vi "Main.vi"() -> ()   [LabVIEW 2013]
uses:
  <vilib>/vision/Image Controls.llb/IMAQ Image.ctl
  <vilib>/Instr/_visa.llb/VISA Flush IO Buffer Mask.ctl
  <vilib>/Instr/_visa.llb/VISA Configure Serial Port (Instr).vi
  <vilib>/vision/NI_Vision_Development_Module.lvlib
panel:
  out "Original Heading Image":T1
  out "Roll Array":dbl[](array[numeric])
  out "Pitch Array":dbl[](array[numeric])
  out "Time for Orientation":dbl[](array[numeric])
  out "Time for Temp":dbl[](array[numeric])
  out "Heater Temp":dbl[](array[numeric])
  out "Temp 2":dbl[](array[numeric])
  out "Temp 1":dbl[](array[numeric])
  out "Start time (minutes)":dbl
  out "error out":errorcluster
  in  "error in (no error)":errorcluster
  in  "Tab Control":T2(tab)
  in  "Yaw":dbl(slide) scale=-180.0..180.0
  in  "Roll":dbl(slide) scale=-10.0..10.0
  in  "Pitch":dbl(slide) scale=-10.0..10.0
  out "Manual Heat Control?":bool
  out "Current Time":timestamp format="%<%I:%M:%S %p>T"
  in  "Command":u16(ring) items=["CUTDOWN"=0, "CHANGE_TRANSMIT_RATE"=1, "TURN_HEATER_ON"=2, "TURN_HEATER_OFF"=3, "MANUAL_HEATER_CONTROL"=4, "GET_INTERIOR_TEMP"=16534, "GET_EXTERIOR_TEMP"=16535, "GET_PRESSURE"=16536, "GET_HUMIDITY"=16537, "GET_PITCH"=16640, "GET_ROLL"=16641, "GET_YAW"=16642, "GET_HEATER_STATUS"=16643]
  in  "Value":u16
  out "Sensor Specifications Exceeded":bool caption="Warning"
  in  "Stop":bool
  in  "Last Recieved Packet":string
  out "Radio Connection Lost":bool caption="Alarm"
  out "Turbulence":bool caption="Warning"
  out "Success?":bool
  in  "Baud Rate":i32=115200
  out "Data Logging OFF":bool caption="Warning"
  in  "Packet Logging File":path
  in  "Log Recieved Packets?":bool=TRUE
  out "Time of Last Recieved Packet":timestamp format="%<%I:%M:%S %p>T"
  out "Heater On?":bool
  out "Yaw":dbl
  out "Roll":dbl
  out "Pitch":dbl
  in  "COM Port":refnum<visa-resource-name>
  in  "Send Command":bool
  out "Response":string
  in  "Interior Temperature 2":dbl(knob) scale=-60.0..40.0
  out "Yaw":T1(plugin-control)
  out "Pitch":dbl(slide) scale=-25.0..25.0
  out "Roll":dbl(slide) scale=-25.0..25.0
  out "Relative Humidity":dbl(knob) scale=0.0..100.0
  out "Atmospheric Pressure":dbl(knob) scale=0.0..15.0
  out "Flight Duration":timestamp format="%<%H:%M:%S>T"
  out "Low Interior Temperature":bool caption="Warning"
  out "Critically Low Interior Temperature":bool caption="Alarm"
  in  "Interior Temperature 1":dbl(knob) scale=-60.0..40.0
  in  "Exterior Temperature":dbl(knob) scale=-60.0..40.0
  in  "Heater Temperature":dbl(knob) scale=-60.0..40.0
  out "Yaw":cluster{"X":dbl, "Y":dbl}[](graph)
  out "Atmospheric Pressure":cluster{"X":dbl, "Y":dbl}[](graph)
  out "Exterior Temperature":cluster{"X":dbl, "Y":dbl}[](graph)
  out "Relative Humidity":cluster{"X":dbl, "Y":dbl}[](graph)
  out "Interior Temperature":cluster{dbl[], dbl[]}[](graph)
  out "Pitch/Roll":cluster{dbl[], dbl[]}[](graph)
  in  "Save Packets":bool
  in  "Packet File":path
  out "Packets Recieved":string
  # "Current Instrument Readings"
  # "Orientation"
  # "Control"
  # "Warnings and Alarms"
  # "Communication"
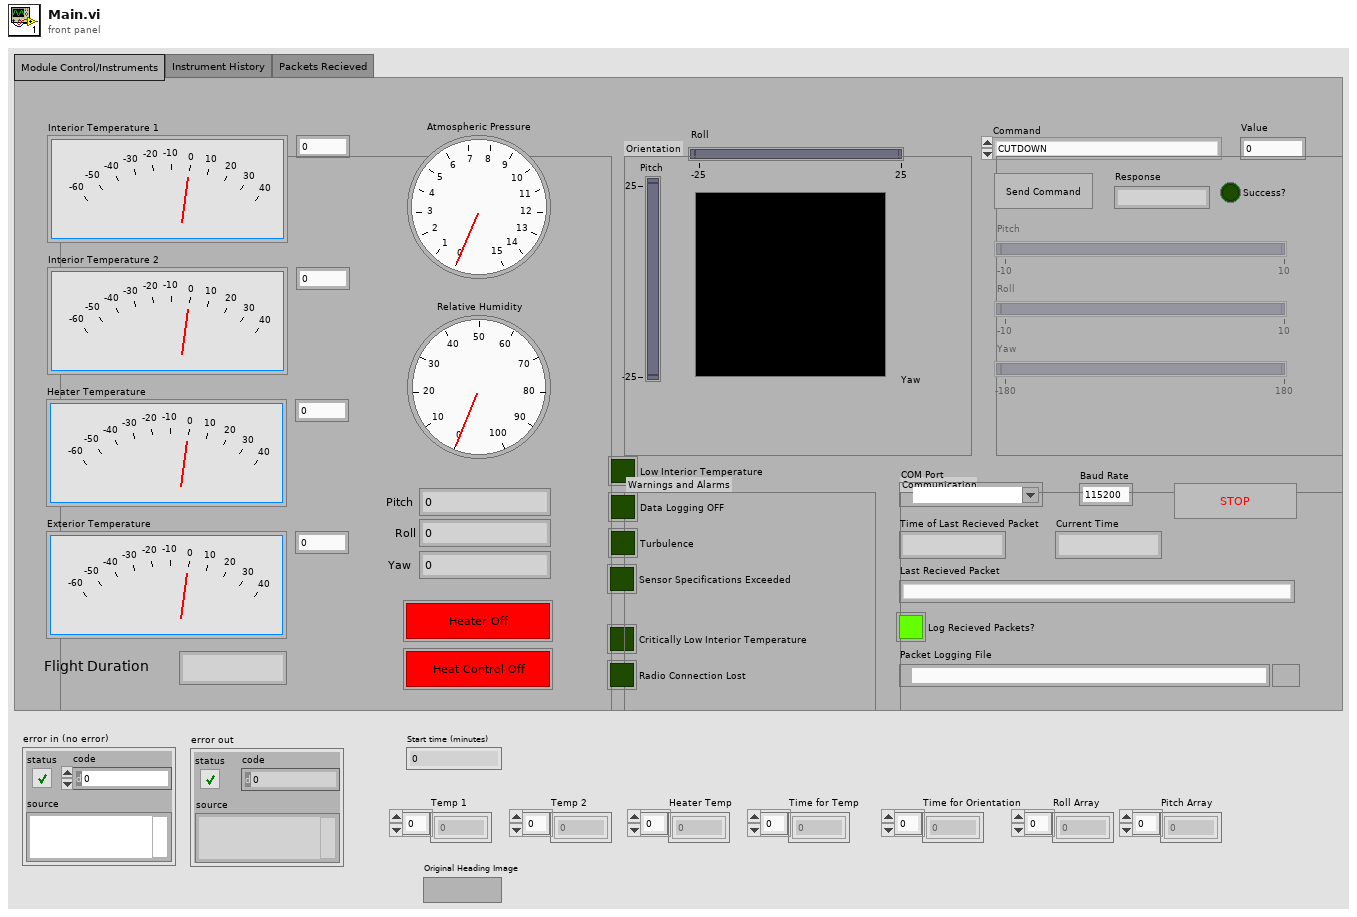
[diagram p1: front panel]
types:
  T1 = typedef "IMAQ Image.ctl" = refnum<image>
  T2 = enum32{"Module Control/Instruments", "Instrument History", "Packets Recieved"}
  T3 = typedef "VISA Flush IO Buffer Mask.ctl" = u16
  T4 = enum16{"open", "replace", "create", "open or create", "replace or create", "replace or create with confirmation"}
  T5 = cluster{"Blue or Luma":u8, "Green or Sat Plane":u8, "Red or Hue Plane":u8, "Alpha":u8}
  T6 = cluster{"Digital Interior Temperature":dbl, "Analog Interior Temperature":dbl, "Heater Temperature":dbl, "Exterior Temperature":dbl, "Humidity":dbl, "Pressure":dbl, "Pitch":dbl, "Roll":dbl, "Yaw":dbl, "Heater On?":bool, "Data Logging?":bool, "Manual Heat Control?":bool, "Turbulence":bool}
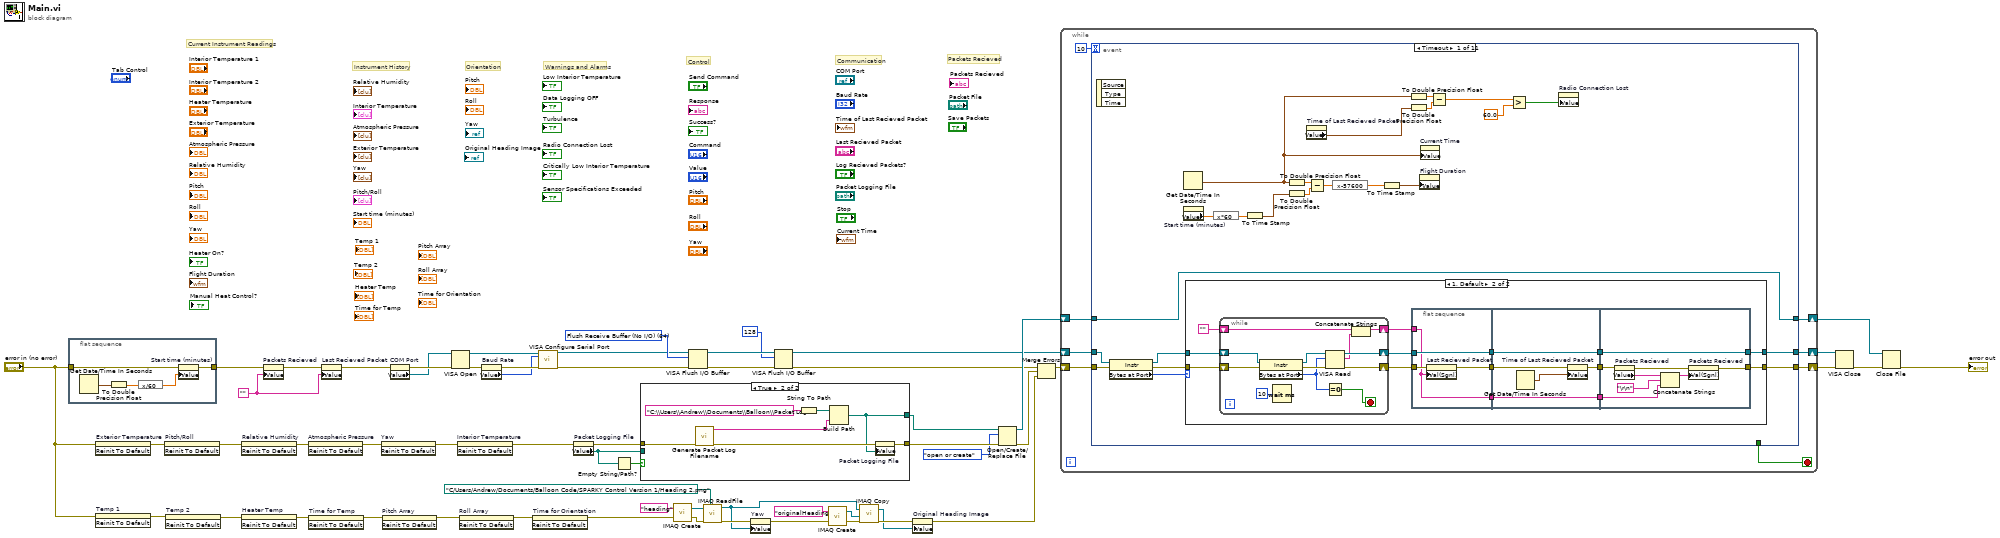
[diagram p0: block diagram]
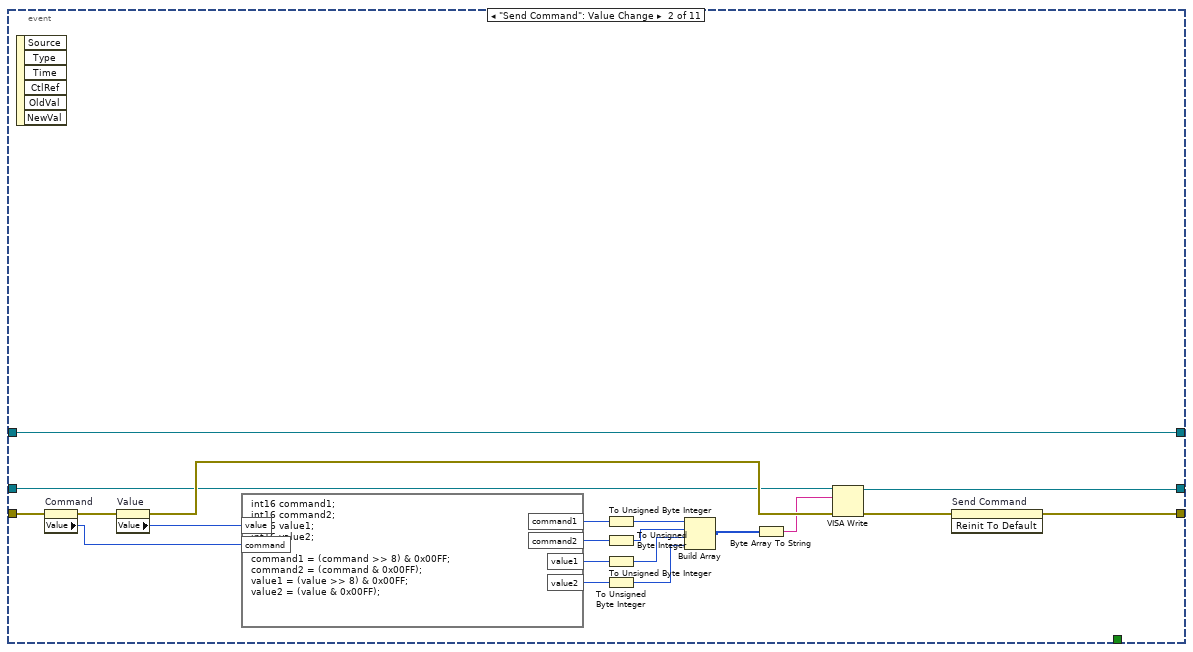
[diagram p4: hidden frame]
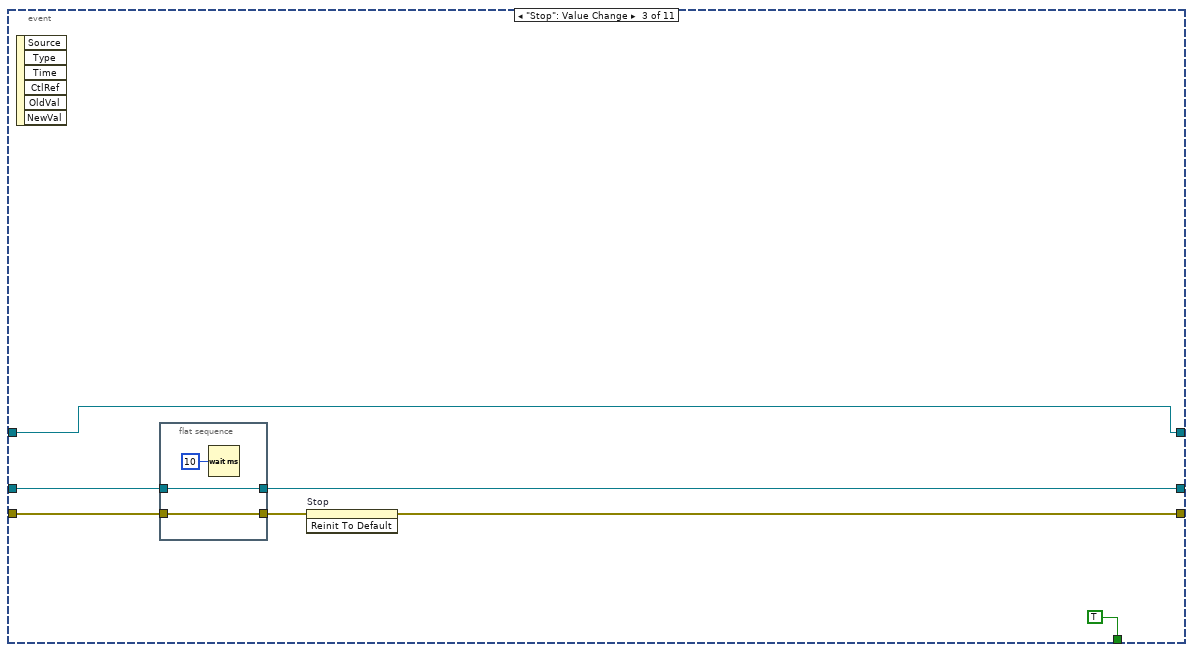
[diagram p5: hidden frame]
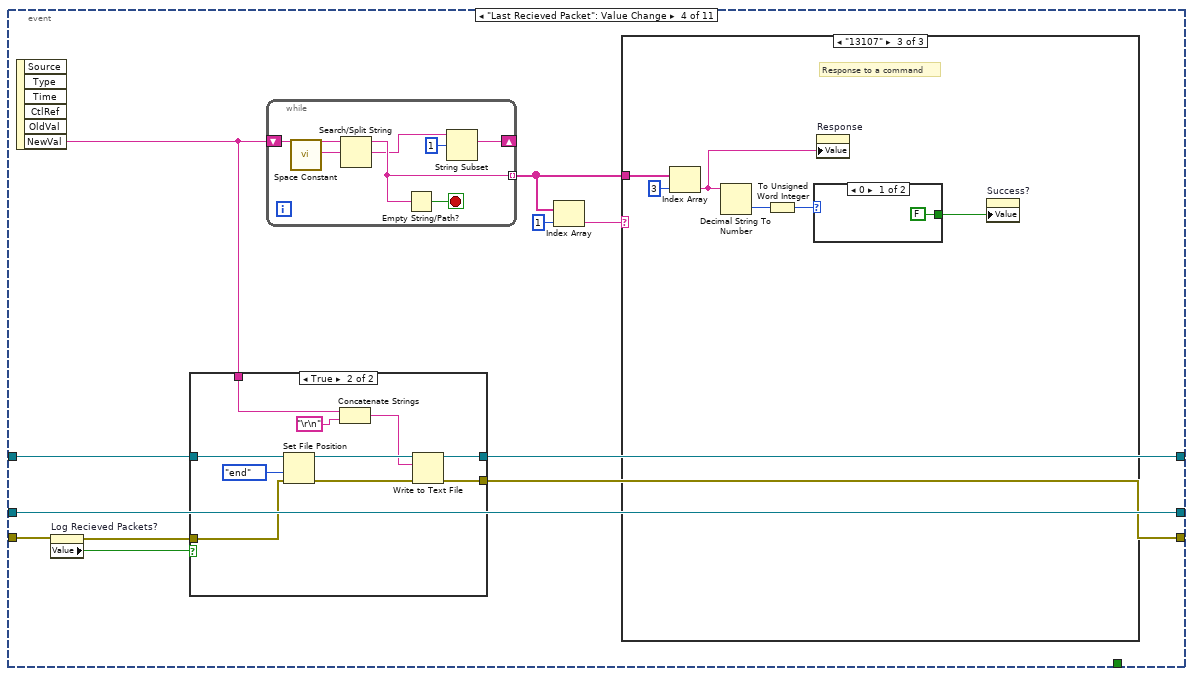
[diagram p6: hidden frame]
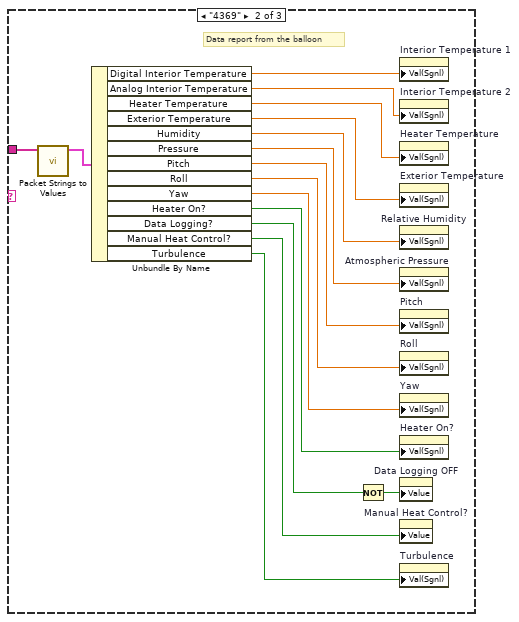
[diagram p8: hidden frame]
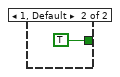
[diagram p9: hidden frame]
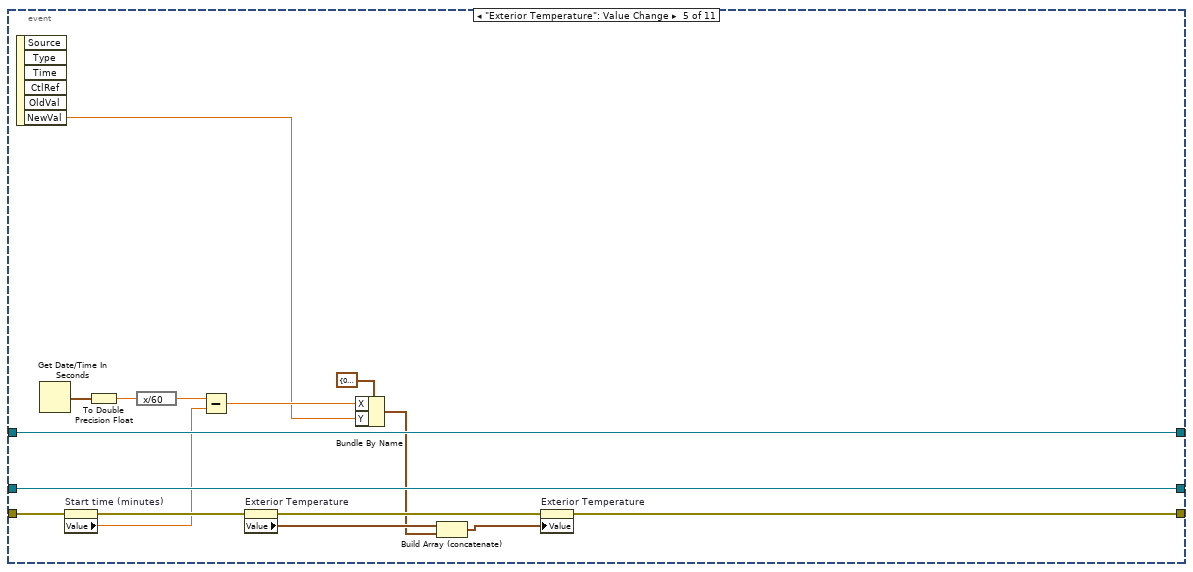
[diagram p11: hidden frame]
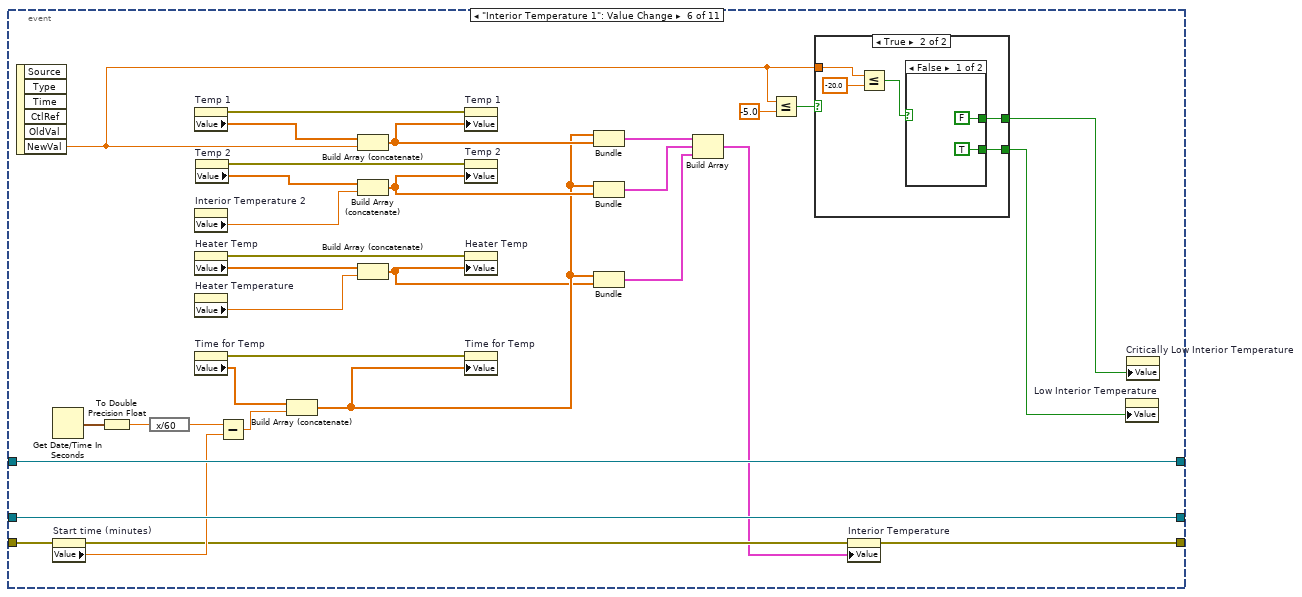
[diagram p12: hidden frame]
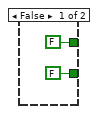
[diagram p13: hidden frame]
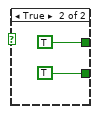
[diagram p14: hidden frame]
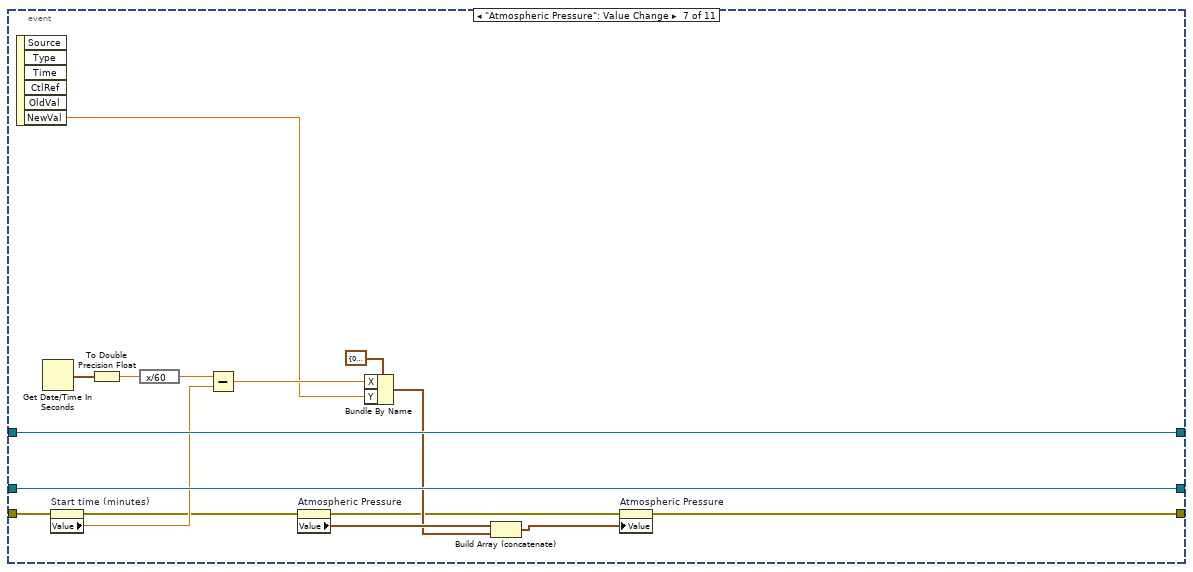
[diagram p15: hidden frame]
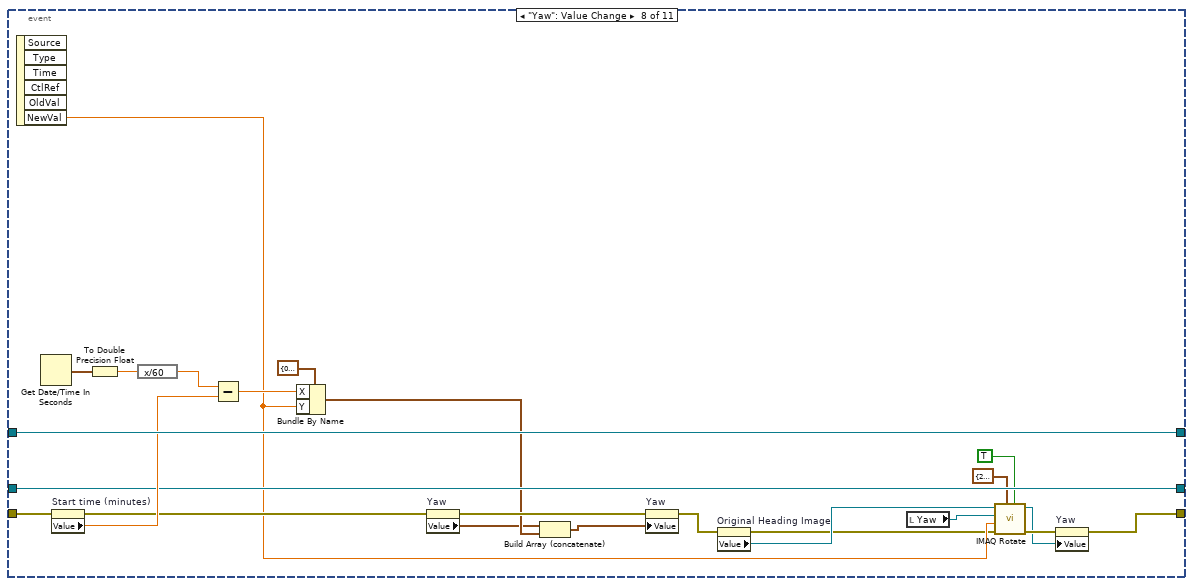
[diagram p16: hidden frame]
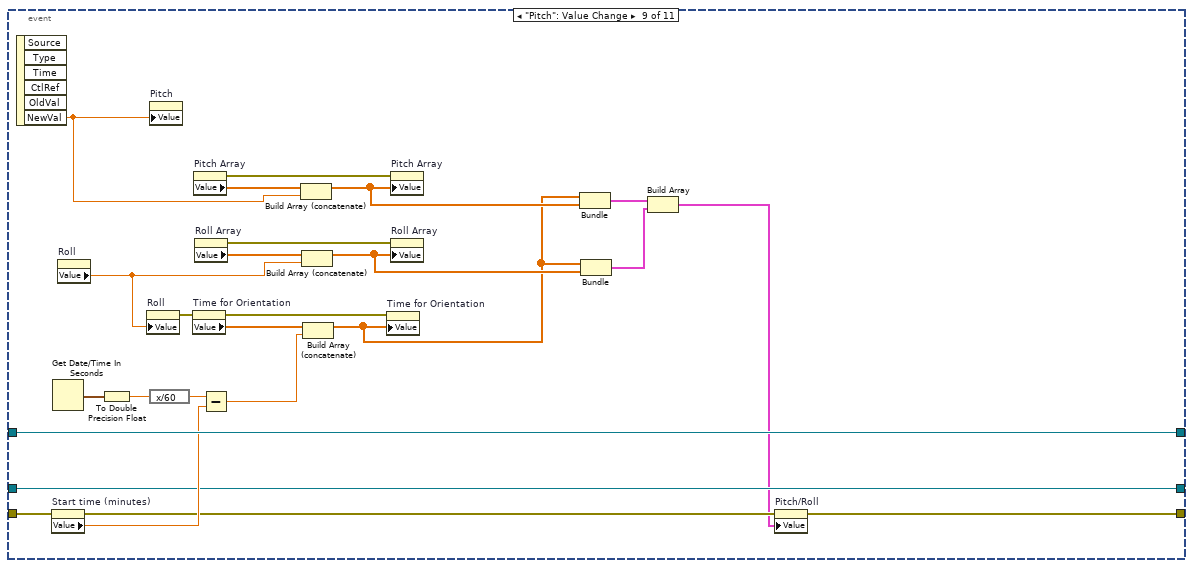
[diagram p17: hidden frame]
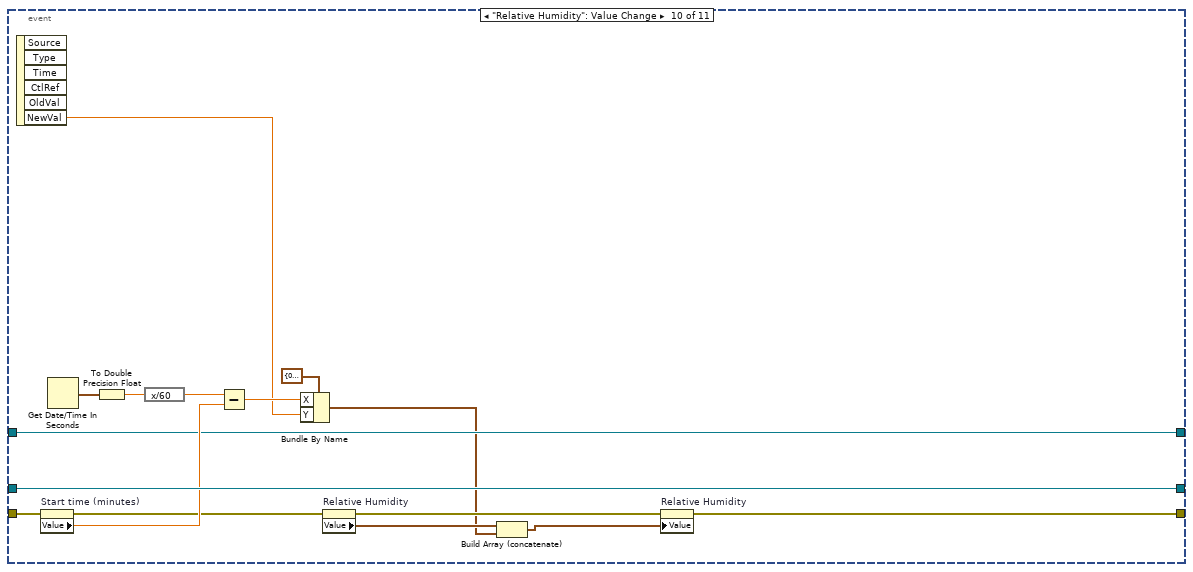
[diagram p18: hidden frame]
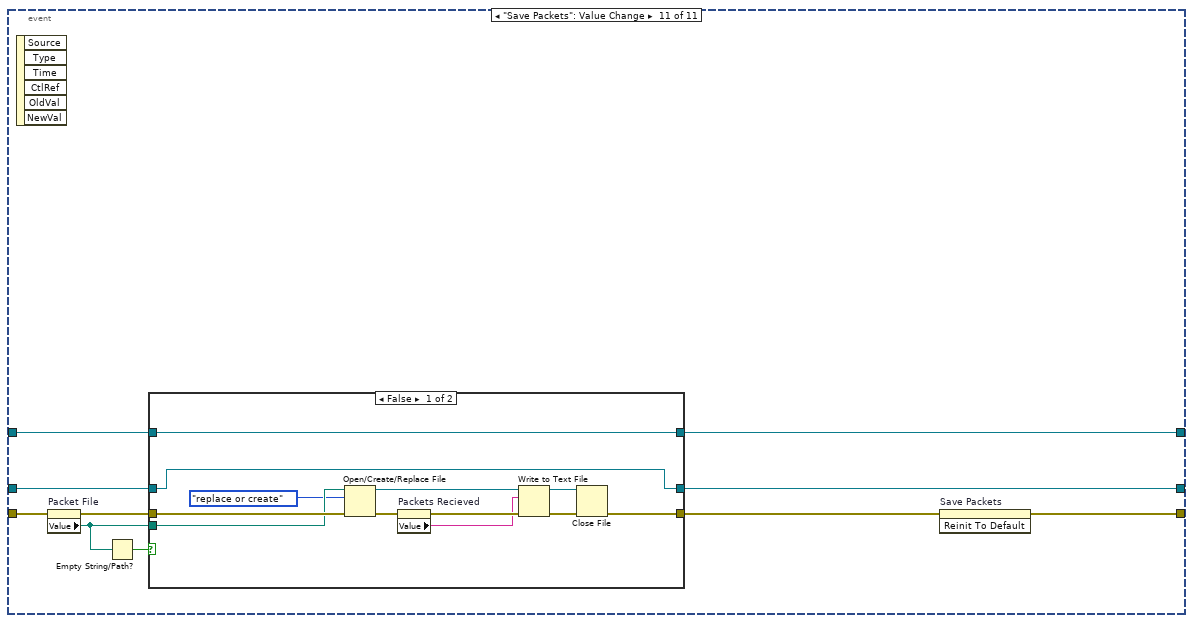
[diagram p19: hidden frame]
diagram:
  w41 = T3 64 items=["Flush Receive Buffer"=16, "Write Transmit Buffer to Device"=32, "Flush Receive Buffer (No I/O)"=64, "Flush Transmit Buffer"=128] ("Mask")
  w30 = ""
  # "Packets Recieved"
  # "Control"
  # "Communication"
  # "Warnings and Alarms"
  # "Orientation"
  # "Current Instrument Readings"
  # "Instrument History"
  n1 = flat-sequence {
    tunnel: "error in (no error)" -> [w61]
    tunnel: [w62] -> w29
    frame #0 {
      n2 = Get Date/Time In Seconds() -> (seconds since 1Jan1904=w64:timestamp)
      n3 = To Double Precision Float(number=w64) -> (double precision float=w63:dbl)
      n4 = expression code="x/60"(w63) -> (w60:dbl)
      n5 = property on="Start time (minutes)" class="DigNum (strict)"(error in=w61, "Value"=w60) -> (error out=w62:errorcluster)  [unwired: 1 in, 1 out]
    }
  }
  n6 = invoke on="Exterior Temperature" class="XYGraph (strict)" method="Reinit To Default"(error in="error in (no error)") -> (error out=w26:errorcluster)  [unwired: 2 in, 2 out]
  n7 = invoke on="Temp 1" class="Arr (strict)" method="Reinit To Default"(error in="error in (no error)") -> (error out=w22:errorcluster)  [unwired: 2 in, 2 out]
  n8 = invoke on="Pitch/Roll" class="XYGraph (strict)" method="Reinit To Default"(error in=w26) -> (error out=w25:errorcluster)  [unwired: 2 in, 2 out]
  n9 = invoke on="Temp 2" class="Arr (strict)" method="Reinit To Default"(error in=w22) -> (error out=w21:errorcluster)  [unwired: 2 in, 2 out]
  n10 = invoke on="Relative Humidity" class="XYGraph (strict)" method="Reinit To Default"(error in=w25) -> (error out=w28:errorcluster)  [unwired: 2 in, 2 out]
  n11 = invoke on="Heater Temp" class="Arr (strict)" method="Reinit To Default"(error in=w21) -> (error out=w20:errorcluster)  [unwired: 2 in, 2 out]
  n12 = property on="Packets Recieved" class="Str"(error in=w29, "Value"=w30) -> (error out=w32:errorcluster)  [unwired: 1 in, 1 out]
  n13 = invoke on="Atmospheric Pressure" class="XYGraph (strict)" method="Reinit To Default"(error in=w28) -> (error out=w27:errorcluster)  [unwired: 2 in, 2 out]
  n14 = invoke on="Time for Temp" class="Arr (strict)" method="Reinit To Default"(error in=w20) -> (error out=w19:errorcluster)  [unwired: 2 in, 2 out]
  n15 = property on="Last Recieved Packet" class="Str"(error in=w32, "Value"=w30) -> (error out=w31:errorcluster)  [unwired: 1 in, 1 out]
  n16 = invoke on="Yaw" class="XYGraph (strict)" method="Reinit To Default"(error in=w27) -> (error out=w23:errorcluster)  [unwired: 2 in, 2 out]
  n17 = invoke on="Pitch Array" class="Arr (strict)" method="Reinit To Default"(error in=w19) -> (error out=w18:errorcluster)  [unwired: 2 in, 2 out]
  n18 = property on="COM Port" class="VISAName"(error in=w31) -> (error out=w54:errorcluster, "Value"=w53:refnum<visa-resource-name>)  [unwired: 1 in, 1 out]
  n19 = VISA Open(error in (no error)=w54, VISA resource name=w53) -> (VISA resource name=w59:refnum<visa-resource-name>, error out=w57:errorcluster)  [unwired: 3 in]
  n20 = invoke on="Interior Temperature" class="XYGraph (strict)" method="Reinit To Default"(error in=w23) -> (error out=w24:errorcluster)  [unwired: 2 in, 2 out]
  n21 = invoke on="Roll Array" class="Arr (strict)" method="Reinit To Default"(error in=w18) -> (error out=w16:errorcluster)  [unwired: 2 in, 2 out]
  n22 = property on="Baud Rate" class="DigNum (strict)"(error in=w57) -> (error out=w56:errorcluster, "Value"=w55:i32)  [unwired: 1 in, 1 out]
  n23 = invoke on="Time for Orientation" class="Arr (strict)" method="Reinit To Default"(error in=w16) -> (error out=w12:errorcluster)  [unwired: 2 in, 2 out]
  n24 = call-poly "VISA Configure Serial Port"("VISA resource name"=w59, "baud rate (9600)"=w55, "error in (no error)"=w56) -> ("VISA resource name out"=w38:refnum<visa-resource-name>, "error out"=w37:errorcluster)  [unwired: 11 in]
  n25 = property on="Packet Logging File" class="Path"(error in=w24) -> (error out=w50:errorcluster, "Value"=w49:path)  [unwired: 1 in, 1 out]
  n26 = Empty String/Path?(string/path=w49) -> (empty?=w51:bool)
  n27 = case shown="True" w51 {
    tunnel: w50 -> [w66 w73]
    tunnel: [w66 w69] -> w48
    tunnel: [w65 w67] -> w43
    tunnel: w49 -> [w65 _]
    frame False {
    }
    frame True {
      n28 = call "Generate Packet Log Filename.vi"("error in (no error)"=w73) -> ("error out"=w68:errorcluster, "Filename"=w70:string)  [unwired: 9 in]
      n29 = String To Path(string="C:\\Users\\Andrew\\Documents\\Balloon\\Packet Logs") -> (path=w72:path)
      n30 = Build Path(base path=w72, name or relative path=w70) -> (appended path=w67:path)
      n31 = property on="Packet Logging File" class="Path"(error in=w68, "Value"=w67) -> (error out=w69:errorcluster)  [unwired: 1 in, 1 out]
    }
  }
  n32 = call "IMAQ Create"("Image Name"="heading", "error in (no error)"=w12) -> ("New Image"=w15:T1, "error out"=w14:errorcluster)  [unwired: 3 in]
  n33 = VISA Flush I/O Buffer(VISA resource name=w38, mask (16)=w41, error in (no error)=w37) -> (VISA resource name out=w40:refnum<visa-resource-name>, error out=w39:errorcluster)
  n34 = call "IMAQ ReadFile"("File Path"=path "C:/Users/Andrew/Documents/Balloon Code/SPARKY Control Version 1/Heading 2.png", "error in (no error)"=w14, "Image"=w15) -> ("error out"=w11:errorcluster, "Image Out"=w5:T1)  [unwired: 4 in, 3 out]
  n35 = property on="Yaw" class="ImageControl"(error in=w11, "Value"=w5) -> (error out=w9:errorcluster)  [unwired: 1 in, 1 out]
  n36 = VISA Flush I/O Buffer(VISA resource name=w40, mask (16)=128, error in (no error)=w39) -> (VISA resource name out=w36:refnum<visa-resource-name>, error out=w35:errorcluster)
  n37 = call "IMAQ Create"("Image Name"="originalHeading", "error in (no error)"=w9) -> ("New Image"=w4:T1, "error out"=w8:errorcluster)  [unwired: 3 in]
  n38 = call "IMAQ Copy"("error in (no error)"=w8, "Image Dst"=w4, "Image Src"=w5) -> ("error out"=w7:errorcluster, "Image Dst Out"=w2:T1)  [unwired: 3 in]
  n39 = property on="Original Heading Image" class="IMAQImage (strict)"(error in=w7, "Value"=w2) -> (error out=w6:errorcluster)  [unwired: 1 in, 1 out]
  n40 = Open/Create/Replace File(file path (use dialog)=w43, error in=w48, operation (0:open)=T4."open or create") -> (refnum out=w42:refnum<file>, error out=w33:errorcluster)  [unwired: 3 in, 1 out]
  n41 = Merge Errors(w35, w33, w6) -> (w34:errorcluster)
  n42 = while {
    shift-right: [w80] -> w58
    shift-left: w34 -> [w81]
    shift-right: [w76] -> w52
    shift-left: w36 -> [w77]
    shift-right: [w74] -> w45
    shift-left: w42 -> [w75]
    stop <- w79 stop-if-true
    n43 = event shown="[0] Timeout" {
      selector: _ -> [_ _ _ _ _ _ _ _ _ _ _]
      dyn-events: _ -> [_ _ _ _ _ _ _ _ _ _ _]
      timeout: 10 -> [_ _ _ _ _ _ _ _ _ _ _]
      tunnel: w81 -> [w104 w167 w171 w186 w241 w282 w308 w333 w358 w374 w384]
      tunnel: [w100 w151 w174 w187 w246 w259 w296 w316 w344 w365 w376] -> w80
      tunnel: [_ _ TRUE _ _ _ _ _ _ _ _] -> w79
      tunnel: w77 -> [w103 w153 w173 w190 w248 w280 w307 w323 w343 w373 w378]
      tunnel: [w98 w169 w172 w190 w248 w280 w307 w323 w343 w373 w377] -> w76
      tunnel: w75 -> [w97 w168 w170 w189 w249 w281 w309 w332 w357 w368 w380]
      tunnel: [w97 w168 w170 w188 w249 w281 w309 w332 w357 w368 w379] -> w74
      event Timeout {
        n44 = event-data() -> ()  [unwired: 1 in, 3 out]
        n45 = property class="Instr"(reference=w103, error in=w104) -> (reference out=w99:refnum<visa-resource-name>, error out=w101:errorcluster, "Bytes at Port"=w102:u32)
        n46 = Get Date/Time In Seconds() -> (seconds since 1Jan1904=w86:timestamp)
        n47 = property on="Start time (minutes)" class="DigNum (strict)"() -> ("Value"=w96:dbl)  [unwired: 2 in, 2 out]
        n48 = case shown="1, Default" w102 {
          tunnel: w101 -> [w105 w111]
          tunnel: [w105 w117] -> w100
          tunnel: w99 -> [w106 w112]
          tunnel: [w106 w118] -> w98
          frame 0 {
          }
          frame 1, Default {
            n49 = while {
              shift-right: [w128] -> w110
              shift-left: w112 -> [w130]
              shift-right: [w127] -> w109
              shift-left: w111 -> [w132]
              shift-right: [w123] -> w107
              shift-left: "" -> [w124]
              stop <- w125 stop-if-true
              n50 = property class="Instr"(reference=w130, error in=w132) -> (reference out=w129:refnum<visa-resource-name>, error out=w131:errorcluster, "Bytes at Port"=w126:u32)
              n51 = Wait (ms)(milliseconds to wait=u32 10) -> ()  [unwired: 1 out]
              n52 = VISA Read(VISA resource name=w129, byte count=w126, error in (no error)=w131) -> (VISA resource name out=w128:refnum<visa-resource-name>, read buffer=w122:string, error out=w127:errorcluster)  [unwired: 1 out]
              n53 = Equal To 0?(x=w126) -> (x = 0?=w125:bool)
              n54 = Concatenate Strings(w124, w122) -> (w123:string)
            }
            n55 = flat-sequence {
              tunnel: w109 -> [w134]
              tunnel: w110 -> [w135]
              tunnel: [w135] -> w120
              tunnel: [w136] -> w119
              tunnel: [w133] -> w113
              tunnel: w107 -> [w133]
              tunnel: w120 -> [w140]
              tunnel: w119 -> [w141]
              tunnel: [w140] -> w116
              tunnel: [w139] -> w115
              tunnel: [w137] -> w114
              tunnel: w113 -> [w137]
              tunnel: [w143] -> w117
              tunnel: [w149] -> w118
              tunnel: w116 -> [w149]
              tunnel: w115 -> [w144]
              tunnel: w114 -> [w142]
              frame #0 {
                n56 = property on="Last Recieved Packet" class="Str"(error in=w134, "Val(Sgnl)"=w133) -> (error out=w136:errorcluster)  [unwired: 1 in, 1 out]
              }
              frame #1 {
                n57 = Get Date/Time In Seconds() -> (seconds since 1Jan1904=w138:timestamp)
                n58 = property on="Time of Last Recieved Packet" class="AbsTime (strict)"(error in=w141, "Value"=w138) -> (error out=w139:errorcluster)  [unwired: 1 in, 1 out]
              }
              frame #2 {
                n59 = property on="Packets Recieved" class="Str"(error in=w144) -> (error out=w147:errorcluster, "Value"=w145:string)  [unwired: 1 in, 1 out]
                n60 = Concatenate Strings(w145, "\r\n", w142) -> (w148:string)
                n61 = property on="Packets Recieved" class="Str"(error in=w147, "Val(Sgnl)"=w148) -> (error out=w143:errorcluster)  [unwired: 1 in, 1 out]
              }
            }
          }
        }
        n62 = expression code="x*60"(w96) -> (w95:dbl)
        n63 = To Time Stamp(1:w95) -> (0:w92:timestamp)
        n64 = To Double Precision Float(number=w86) -> (double precision float=w93:dbl)
        n65 = To Double Precision Float(number=w92) -> (double precision float=w91:dbl)
        n66 = property on="Time of Last Recieved Packet" class="AbsTime (strict)"() -> ("Value"=w85:timestamp)  [unwired: 2 in, 2 out]
        n67 = Subtract(x=w93, y=w91) -> (x-y=w90:dbl)
        n68 = expression code="x-57600"(w90) -> (w89:dbl)
        n69 = To Time Stamp(1:w89) -> (0:w94:timestamp)
        n70 = To Double Precision Float(number=w86) -> (double precision float=w88:dbl)
        n71 = To Double Precision Float(number=w85) -> (double precision float=w87:dbl)
        n72 = property on="Flight Duration" class="AbsTime (strict)"("Value"=w94) -> ()  [unwired: 2 in, 2 out]
        n73 = property on="Current Time" class="AbsTime (strict)"("Value"=w86) -> ()  [unwired: 2 in, 2 out]
        n74 = Subtract(x=w88, y=w87) -> (x-y=w82:dbl)
        n75 = Greater?(x=w82, y=60.0) -> (0:w83:bool)
        n76 = property on="Radio Connection Lost" class="Bool (strict)"("Value"=w83) -> ()  [unwired: 2 in, 2 out]
      }
      event "Send Command": Value Change {
        n77 = event-data() -> ()  [unwired: 1 in, 6 out]
        n78 = property on="Command" class="Ring (strict)"(error in=w167) -> (error out=w166:errorcluster, "Value"=w165:u16)  [unwired: 1 in, 1 out]
        n79 = property on="Value" class="DigNum (strict)"(error in=w166) -> (error out=w155:errorcluster, "Value"=w164:u16)  [unwired: 1 in, 1 out]
        n80 = formula code="int16 command1;\nint16 command2;\nint16 value1;\nint16 value2;\n\ncommand1 = (command >> 8) & 0x00FF;\ncommand2 = (command & 0x00FF);\nvalue1 = (value >> 8) & 0x00FF;\nvalue2 = (value & 0x00FF);"("command"=w165, "value"=w164) -> ("command1"=w162:i16, "command2"=w161:i16, "value1"=w160:i16, "value2"=w159:i16)
        n81 = To Unsigned Byte Integer(number=w162) -> (unsigned 8bit integer=w163:u8)
        n82 = To Unsigned Byte Integer(number=w161) -> (unsigned 8bit integer=w158:u8)
        n83 = To Unsigned Byte Integer(number=w160) -> (unsigned 8bit integer=w157:u8)
        n84 = To Unsigned Byte Integer(number=w159) -> (unsigned 8bit integer=w156:u8)
        n85 = Build Array(w163, w158, w157, w156) -> (w150:u8[])
        n86 = Byte Array To String(unsigned byte array=w150) -> (string=w154:string)
        n87 = VISA Write(VISA resource name=w153, write buffer=w154, error in (no error)=w155) -> (VISA resource name out=w169:refnum<visa-resource-name>, error out=w152:errorcluster)  [unwired: 1 out]
        n88 = invoke on="Send Command" class="Bool" method="Reinit To Default"(error in=w152) -> (error out=w151:errorcluster)  [unwired: 2 in, 2 out]
      }
      event "Stop": Value Change {
        n89 = event-data() -> ()  [unwired: 1 in, 6 out]
        n90 = flat-sequence {
          tunnel: w171 -> [w178]
          tunnel: [w178] -> w175
          tunnel: w173 -> [w177]
          tunnel: [w177] -> w172
          frame #0 {
            n91 = Wait (ms)(milliseconds to wait=u32 10) -> ()  [unwired: 1 out]
          }
        }
        n92 = invoke on="Stop" class="Bool" method="Reinit To Default"(error in=w175) -> (error out=w174:errorcluster)  [unwired: 2 in, 2 out]
      }
      event "Last Recieved Packet": Value Change {
        n93 = event-data() -> ("NewVal"=w183:string)  [unwired: 1 in, 5 out]
        n94 = property on="Log Recieved Packets?" class="Bool (strict)"(error in=w186) -> (error out=w185:errorcluster, "Value"=w184:bool)  [unwired: 1 in, 1 out]
        n95 = case shown="True" w184 {
          tunnel: w189 -> [w223 w230]
          tunnel: [w223 w229] -> w188
          tunnel: [w222 w228] -> w187
          tunnel: w185 -> [w222 w227]
          tunnel: w183 -> [_ w226]
          frame False {
          }
          frame True {
            n96 = Set File Position(refnum=w230, from (0:start)=enum16{"start", "end", "current"}."end", error in=w227) -> (refnum out=w231:refnum<file>, error out=w232:errorcluster)  [unwired: 1 in]
            n97 = Concatenate Strings(w226, "\r\n") -> (w224:string)
            n98 = Write to Text File(file (use dialog)=w231, text=w224, error in=w232) -> (refnum out=w229:refnum<file>, error out=w228:errorcluster)  [unwired: 1 in, 1 out]
          }
        }
        n99 = while {
          shift-right: [w215] -> _
          shift-left: w183 -> [w220]
          tunnel: [w218] -> w180 mode=indexing
          stop <- w221 stop-if-true
          n100 = call <vilib>:"Space Constant.vi"() -> ("String"=w219:string)
          n101 = Search/Split String(string=w220, search string/char (-)=w219) -> (substring before match=w218:string, match + rest of string=w217:string)  [unwired: 1 in, 1 out]
          n102 = Empty String/Path?(string/path=w218) -> (empty?=w221:bool)
          n103 = String Subset(string=w217, offset (0)=1) -> (substring=w215:string)  [unwired: 1 in]
        }
        n104 = Index Array(array=w180, index=1) -> (element=w181:string)
        n105 = case shown="\"13107\"" w181 {
          tunnel: w180 -> [_ w206 w212]
          frame Default {
          }
          frame "4369" {
            # "Data report from the balloon"
            n106 = call "Packet Strings to Values.vi"("Pakcet Values"=w206) -> ("Data Report"=w205:T6)  [unwired: 10 in]
            n107 = Unbundle By Name(w205) -> ("Digital Interior Temperature"=w204:dbl, "Analog Interior Temperature"=w203:dbl, "Heater Temperature"=w202:dbl, "Exterior Temperature"=w201:dbl, "Humidity"=w200:dbl, "Pressure"=w199:dbl, "Pitch"=w198:dbl, "Roll"=w197:dbl, "Yaw"=w196:dbl, "Heater On?"=w195:bool, "Data Logging?"=w192:bool, "Manual Heat Control?"=w194:bool, "Turbulence"=w191:bool)
            n108 = Not(x=w192) -> (.not. x?=w193:bool)
            n109 = property on="Interior Temperature 1" class="Knob (strict)"("Val(Sgnl)"=w204) -> ()  [unwired: 2 in, 2 out]
            n110 = property on="Interior Temperature 2" class="Knob (strict)"("Val(Sgnl)"=w203) -> ()  [unwired: 2 in, 2 out]
            n111 = property on="Heater Temperature" class="Knob (strict)"("Val(Sgnl)"=w202) -> ()  [unwired: 2 in, 2 out]
            n112 = property on="Exterior Temperature" class="Knob (strict)"("Val(Sgnl)"=w201) -> ()  [unwired: 2 in, 2 out]
            n113 = property on="Relative Humidity" class="Knob (strict)"("Val(Sgnl)"=w200) -> ()  [unwired: 2 in, 2 out]
            n114 = property on="Atmospheric Pressure" class="Knob (strict)"("Val(Sgnl)"=w199) -> ()  [unwired: 2 in, 2 out]
            n115 = property on="Pitch" class="DigNum (strict)"("Val(Sgnl)"=w198) -> ()  [unwired: 2 in, 2 out]
            n116 = property on="Roll" class="DigNum (strict)"("Val(Sgnl)"=w197) -> ()  [unwired: 2 in, 2 out]
            n117 = property on="Yaw" class="DigNum (strict)"("Val(Sgnl)"=w196) -> ()  [unwired: 2 in, 2 out]
            n118 = property on="Heater On?" class="Bool (strict)"("Val(Sgnl)"=w195) -> ()  [unwired: 2 in, 2 out]
            n119 = property on="Data Logging OFF" class="Bool (strict)"("Value"=w193) -> ()  [unwired: 2 in, 2 out]
            n120 = property on="Manual Heat Control?" class="Bool (strict)"("Value"=w194) -> ()  [unwired: 2 in, 2 out]
            n121 = property on="Turbulence" class="Bool (strict)"("Val(Sgnl)"=w191) -> ()  [unwired: 2 in, 2 out]
          }
          frame "13107" {
            # "Response to a command"
            n122 = Index Array(array=w212, index=3) -> (element=w207:string)
            n123 = Decimal String To Number(string=w207) -> (number=w210:i32)  [unwired: 2 in, 1 out]
            n124 = To Unsigned Word Integer(number=w210) -> (unsigned 16bit integer=w209:u16)
            n125 = case shown="0" w209 {
              tunnel: [FALSE TRUE] -> w208
              frame 0 {
              }
              frame 1, Default {
              }
            }
            n126 = property on="Response" class="Str"("Value"=w207) -> ()  [unwired: 2 in, 2 out]
            n127 = property on="Success?" class="Bool (strict)"("Value"=w208) -> ()  [unwired: 2 in, 2 out]
          }
        }
      }
      event "Exterior Temperature": Value Change {
        n128 = event-data() -> ("NewVal"=w236:dbl)  [unwired: 1 in, 5 out]
        n129 = Get Date/Time In Seconds() -> (seconds since 1Jan1904=w242:timestamp)
        n130 = property on="Start time (minutes)" class="DigNum (strict)"(error in=w241) -> (error out=w240:errorcluster, "Value"=w238:dbl)  [unwired: 1 in, 1 out]
        n131 = To Double Precision Float(number=w242) -> (double precision float=w243:dbl)
        n132 = expression code="x/60"(w243) -> (w239:dbl)
        n133 = Subtract(x=w239, y=w238) -> (x-y=w237:dbl)
        n134 = property on="Exterior Temperature" class="XYGraph (strict)"(error in=w240) -> (error out=w247:errorcluster, "Value"=w245:cluster{"X":dbl, "Y":dbl}[])  [unwired: 1 in, 1 out]
        n135 = Bundle By Name(cluster=cluster{"X":dbl, "Y":dbl} {"X"=0.0, "Y"=0.0} ("element"), "X"=w237, "Y"=w236) -> (w235:cluster{"X":dbl, "Y":dbl})
        n136 = Build Array (concatenate)(w245, w235) -> (w234:cluster{"X":dbl, "Y":dbl}[])
        n137 = property on="Exterior Temperature" class="XYGraph (strict)"(error in=w247, "Value"=w234) -> (error out=w246:errorcluster)  [unwired: 1 in, 1 out]
      }
      event "Interior Temperature 1": Value Change {
        n138 = event-data() -> ("NewVal"=w252:dbl)  [unwired: 1 in, 5 out]
        n139 = Get Date/Time In Seconds() -> (seconds since 1Jan1904=w278:timestamp)
        n140 = property on="Start time (minutes)" class="DigNum (strict)"(error in=w282) -> (error out=w261:errorcluster, "Value"=w276:dbl)  [unwired: 1 in, 1 out]
        n141 = To Double Precision Float(number=w278) -> (double precision float=w277:dbl)
        n142 = expression code="x/60"(w277) -> (w279:dbl)
        n143 = property on="Temp 1" class="Arr (strict)"() -> (error out=w267:errorcluster, "Value"=w270:dbl[])  [unwired: 2 in, 1 out]
        n144 = property on="Interior Temperature 2" class="Knob (strict)"() -> ("Value"=w272:dbl)  [unwired: 2 in, 2 out]
        n145 = property on="Heater Temp" class="Arr (strict)"() -> (error out=w265:errorcluster, "Value"=w268:dbl[])  [unwired: 2 in, 1 out]
        n146 = property on="Heater Temperature" class="Knob (strict)"() -> ("Value"=w271:dbl)  [unwired: 2 in, 2 out]
        n147 = property on="Time for Temp" class="Arr (strict)"() -> (error out=w273:errorcluster, "Value"=w274:dbl[])  [unwired: 2 in, 1 out]
        n148 = property on="Temp 2" class="Arr (strict)"() -> (error out=w266:errorcluster, "Value"=w269:dbl[])  [unwired: 2 in, 1 out]
        n149 = Subtract(x=w279, y=w276) -> (x-y=w275:dbl)
        n150 = Build Array (concatenate)(w274, w275) -> (w256:dbl[])
        n151 = Build Array (concatenate)(w270, w252) -> (w258:dbl[])
        n152 = Build Array (concatenate)(w269, w272) -> (w257:dbl[])
        n153 = Build Array (concatenate)(w268, w271) -> (w255:dbl[])
        n154 = property on="Temp 1" class="Arr (strict)"(error in=w267, "Value"=w258) -> ()  [unwired: 1 in, 2 out]
        n155 = property on="Temp 2" class="Arr (strict)"(error in=w266, "Value"=w257) -> ()  [unwired: 1 in, 2 out]
        n156 = property on="Heater Temp" class="Arr (strict)"(error in=w265, "Value"=w255) -> ()  [unwired: 1 in, 2 out]
        n157 = property on="Time for Temp" class="Arr (strict)"(error in=w273, "Value"=w256) -> ()  [unwired: 1 in, 2 out]
        n158 = Bundle(w256, w258) -> (w264:cluster{dbl[], dbl[]})  [unwired: 1 in]
        n159 = Bundle(w256, w257) -> (w263:cluster{dbl[], dbl[]})  [unwired: 1 in]
        n160 = Bundle(w256, w255) -> (w262:cluster{dbl[], dbl[]})  [unwired: 1 in]
        n161 = Build Array(w264, w263, w262) -> (w260:cluster{dbl[], dbl[]}[])
        n162 = Less Or Equal?(x=w252, y=-5.0) -> (x <= y?=w253:bool)
        n163 = case shown="True" w253 {
          tunnel: w252 -> [_ w288]
          tunnel: [FALSE w286] -> w251
          tunnel: [FALSE w285] -> w250
          frame False {
          }
          frame True {
            n164 = Less Or Equal?(x=w288, y=-20.0) -> (x <= y?=w287:bool)
            n165 = case shown="False" w287 {
              tunnel: [FALSE TRUE] -> w286
              tunnel: [TRUE TRUE] -> w285
              frame False {
              }
              frame True {
              }
            }
          }
        }
        n166 = property on="Interior Temperature" class="XYGraph (strict)"(error in=w261, "Value"=w260) -> (error out=w259:errorcluster)  [unwired: 1 in, 1 out]
        n167 = property on="Low Interior Temperature" class="Bool (strict)"("Value"=w250) -> ()  [unwired: 2 in, 2 out]
        n168 = property on="Critically Low Interior Temperature" class="Bool (strict)"("Value"=w251) -> ()  [unwired: 2 in, 2 out]
      }
      event "Atmospheric Pressure": Value Change {
        n169 = event-data() -> ("NewVal"=w294:dbl)  [unwired: 1 in, 5 out]
        n170 = Get Date/Time In Seconds() -> (seconds since 1Jan1904=w306:timestamp)
        n171 = property on="Start time (minutes)" class="DigNum (strict)"(error in=w308) -> (error out=w301:errorcluster, "Value"=w303:dbl)  [unwired: 1 in, 1 out]
        n172 = To Double Precision Float(number=w306) -> (double precision float=w305:dbl)
        n173 = expression code="x/60"(w305) -> (w304:dbl)
        n174 = Subtract(x=w304, y=w303) -> (x-y=w295:dbl)
        n175 = property on="Atmospheric Pressure" class="XYGraph (strict)"(error in=w301) -> (error out=w298:errorcluster, "Value"=w300:cluster{"X":dbl, "Y":dbl}[])  [unwired: 1 in, 1 out]
        n176 = Bundle By Name(cluster=cluster{"X":dbl, "Y":dbl} {"X"=0.0, "Y"=0.0} ("element"), "X"=w295, "Y"=w294) -> (w299:cluster{"X":dbl, "Y":dbl})
        n177 = Build Array (concatenate)(w300, w299) -> (w297:cluster{"X":dbl, "Y":dbl}[])
        n178 = property on="Atmospheric Pressure" class="XYGraph (strict)"(error in=w298, "Value"=w297) -> (error out=w296:errorcluster)  [unwired: 1 in, 1 out]
      }
      event "Yaw": Value Change {
        n179 = event-data() -> ("NewVal"=w312:dbl)  [unwired: 1 in, 5 out]
        n180 = Get Date/Time In Seconds() -> (seconds since 1Jan1904=w329:timestamp)
        n181 = property on="Start time (minutes)" class="DigNum (strict)"(error in=w333) -> (error out=w325:errorcluster, "Value"=w331:dbl)  [unwired: 1 in, 1 out]
        n182 = To Double Precision Float(number=w329) -> (double precision float=w330:dbl)
        n183 = expression code="x/60"(w330) -> (w328:dbl)
        n184 = Subtract(x=w328, y=w331) -> (x-y=w326:dbl)
        n185 = Bundle By Name(cluster=cluster{"X":dbl, "Y":dbl} {"X"=0.0, "Y"=0.0} ("element"), "X"=w326, "Y"=w312) -> (w322:cluster{"X":dbl, "Y":dbl})
        n186 = property on="Yaw" class="XYGraph (strict)"(error in=w325) -> (error out=w324:errorcluster, "Value"=w321:cluster{"X":dbl, "Y":dbl}[])  [unwired: 1 in, 1 out]
        n187 = Build Array (concatenate)(w321, w322) -> (w320:cluster{"X":dbl, "Y":dbl}[])
        n188 = property on="Yaw" class="XYGraph (strict)"(error in=w324, "Value"=w320) -> (error out=w319:errorcluster)  [unwired: 1 in, 1 out]
        n189 = property on="Original Heading Image" class="IMAQImage (strict)"(error in=w319) -> (error out=w311:errorcluster, "Value"=w315:T1)  [unwired: 1 in, 1 out]
        n190 = local read "Yaw"() -> (w310:T1)
        n191 = call "IMAQ Rotate"("Maintain Size"=TRUE, "Color Replace Value"=T5 {"Blue or Luma"=255, "Green or Sat Plane"=255, "Red or Hue Plane"=255, "Alpha"=0}, "error in (no error)"=w311, "Angle (degrees)"=w312, "Image Dst"=w310, "Image Src"=w315) -> ("error out"=w318:errorcluster, "Image Dst Out"=w317:T1)  [unwired: 4 in]
        n192 = property on="Yaw" class="ImageControl"(error in=w318, "Value"=w317) -> (error out=w316:errorcluster)  [unwired: 1 in, 1 out]
      }
      event "Pitch": Value Change {
        n193 = event-data() -> ("NewVal"=w336:dbl)  [unwired: 1 in, 5 out]
        n194 = property on="Start time (minutes)" class="DigNum (strict)"(error in=w358) -> (error out=w345:errorcluster, "Value"=w353:dbl)  [unwired: 1 in, 1 out]
        n195 = Get Date/Time In Seconds() -> (seconds since 1Jan1904=w355:timestamp)
        n196 = property on="Roll" class="DigNum (strict)"() -> ("Value"=w334:dbl)  [unwired: 2 in, 2 out]
        n197 = To Double Precision Float(number=w355) -> (double precision float=w356:dbl)
        n198 = property on="Roll" class="Slide (strict)"("Value"=w334) -> (error out=w335:errorcluster)  [unwired: 2 in, 1 out]
        n199 = property on="Pitch" class="Slide (strict)"("Value"=w336) -> ()  [unwired: 2 in, 2 out]
        n200 = expression code="x/60"(w356) -> (w354:dbl)
        n201 = property on="Time for Orientation" class="Arr (strict)"(error in=w335) -> (error out=w352:errorcluster, "Value"=w351:dbl[])  [unwired: 1 in, 1 out]
        n202 = property on="Pitch Array" class="Arr (strict)"() -> (error out=w349:errorcluster, "Value"=w346:dbl[])  [unwired: 2 in, 1 out]
        n203 = property on="Roll Array" class="Arr (strict)"() -> (error out=w348:errorcluster, "Value"=w347:dbl[])  [unwired: 2 in, 1 out]
        n204 = Subtract(x=w354, y=w353) -> (x-y=w350:dbl)
        n205 = Build Array (concatenate)(w346, w336) -> (w342:dbl[])
        n206 = Build Array (concatenate)(w347, w334) -> (w341:dbl[])
        n207 = Build Array (concatenate)(w351, w350) -> (w340:dbl[])
        n208 = property on="Time for Orientation" class="Arr (strict)"(error in=w352, "Value"=w340) -> ()  [unwired: 1 in, 2 out]
        n209 = property on="Pitch Array" class="Arr (strict)"(error in=w349, "Value"=w342) -> ()  [unwired: 1 in, 2 out]
        n210 = property on="Roll Array" class="Arr (strict)"(error in=w348, "Value"=w341) -> ()  [unwired: 1 in, 2 out]
        n211 = Bundle(w340, w342) -> (w339:cluster{dbl[], dbl[]})  [unwired: 1 in]
        n212 = Bundle(w340, w341) -> (w338:cluster{dbl[], dbl[]})  [unwired: 1 in]
        n213 = Build Array(w339, w338) -> (w337:cluster{dbl[], dbl[]}[])
        n214 = property on="Pitch/Roll" class="XYGraph (strict)"(error in=w345, "Value"=w337) -> (error out=w344:errorcluster)  [unwired: 1 in, 1 out]
      }
      event "Relative Humidity": Value Change {
        n215 = event-data() -> ("NewVal"=w360:dbl)  [unwired: 1 in, 5 out]
        n216 = property on="Start time (minutes)" class="DigNum (strict)"(error in=w374) -> (error out=w367:errorcluster, "Value"=w369:dbl)  [unwired: 1 in, 1 out]
        n217 = Get Date/Time In Seconds() -> (seconds since 1Jan1904=w371:timestamp)
        n218 = To Double Precision Float(number=w371) -> (double precision float=w372:dbl)
        n219 = expression code="x/60"(w372) -> (w370:dbl)
        n220 = Subtract(x=w370, y=w369) -> (x-y=w361:dbl)
        n221 = Bundle By Name(cluster=cluster{"X":dbl, "Y":dbl} {"X"=0.0, "Y"=0.0} ("element"), "X"=w361, "Y"=w360) -> (w359:cluster{"X":dbl, "Y":dbl})
        n222 = property on="Relative Humidity" class="XYGraph (strict)"(error in=w367) -> (error out=w366:errorcluster, "Value"=w364:cluster{"X":dbl, "Y":dbl}[])  [unwired: 1 in, 1 out]
        n223 = Build Array (concatenate)(w364, w359) -> (w363:cluster{"X":dbl, "Y":dbl}[])
        n224 = property on="Relative Humidity" class="XYGraph (strict)"(error in=w366, "Value"=w363) -> (error out=w365:errorcluster)  [unwired: 1 in, 1 out]
      }
      event "Save Packets": Value Change {
        n225 = event-data() -> ()  [unwired: 1 in, 6 out]
        n226 = property on="Packet File" class="Path"(error in=w384) -> (error out=w383:errorcluster, "Value"=w381:path)  [unwired: 1 in, 1 out]
        n227 = Empty String/Path?(string/path=w381) -> (empty?=w382:bool)
        n228 = case shown="False" w382 {
          tunnel: w383 -> [w396 w399]
          tunnel: w381 -> [w395 _]
          tunnel: [w387 w399] -> w375
          tunnel: w380 -> [w386 w397]
          tunnel: [w386 w397] -> w379
          tunnel: w378 -> [w385 w398]
          tunnel: [w385 w398] -> w377
          frame False {
            n229 = Open/Create/Replace File(file path (use dialog)=w395, error in=w396, operation (0:open)=T4."replace or create") -> (refnum out=w390:refnum<file>, error out=w393:errorcluster)  [unwired: 3 in, 1 out]
            n230 = property on="Packets Recieved" class="Str"(error in=w393) -> (error out=w392:errorcluster, "Value"=w391:string)  [unwired: 1 in, 1 out]
            n231 = Write to Text File(file (use dialog)=w390, text=w391, error in=w392) -> (refnum out=w388:refnum<file>, error out=w389:errorcluster)  [unwired: 1 in, 1 out]
            n232 = Close File(refnum=w388, error in=w389) -> (error out=w387:errorcluster)  [unwired: 1 out]
          }
          frame True {
          }
        }
        n233 = invoke on="Save Packets" class="Bool" method="Reinit To Default"(error in=w375) -> (error out=w376:errorcluster)  [unwired: 2 in, 2 out]
      }
    }
  }
  n234 = VISA Close(VISA resource name=w52, error in (no error)=w58) -> (error out=w46:errorcluster)
  n235 = Close File(refnum=w45, error in=w46) -> (error out=→"error out":errorcluster)  [unwired: 1 out]
